vi "LVObject to JSON - Serializable Class - Returns JSON String.vi"() -> ()   [LabVIEW 2017, in "JSON Serializable Serializer Tests.lvlib"]
uses:
  JSON Serializable Serializer Tests.lvlib
  JSON Serializable Serializer/JSON Serializable Serializer.lvclass
  <vilib>/addons/_JKI Toolkits/Caraya/classes/Assert/Assert Equal Value_Variant.vi
  <vilib>/addons/_JKI Toolkits/Caraya/classes/Test/Test.lvclass
  <vilib>/addons/_JKI Toolkits/Caraya/classes/Assert/Assert.lvclass
  Mock JSON Serializable/Mock JSON Serializable.lvclass
panel:
  out "error out":errorcluster
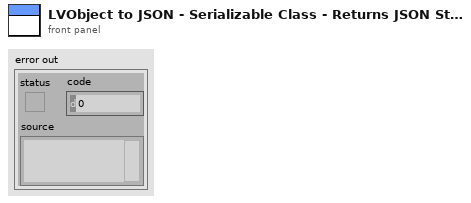
[diagram p1: front panel]
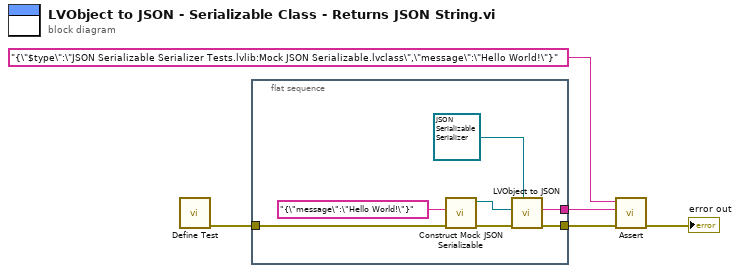
[diagram p0: block diagram]
diagram:
  n1 = call <vilib>:"Define Test.vi"() -> ("error out"=w3:errorcluster)  [unwired: 11 in]
  n2 = flat-sequence {
    tunnel: [w9] -> w5
    tunnel: [w10] -> w4
    tunnel: w3 -> [w11]
    frame #0 {
      n3 = call "Construct Mock JSON Serializable.vi"("error in (no error)"=w11, "To JSON <JSON> (\"{}\")"="{\"message\":\"Hello World!\"}" ("<JSON> (\"{}\")")) -> ("error out"=w8:errorcluster, "Mock JSON Serializable"=w7:refnum<class "Mock JSON Serializable.lvclass">)  [unwired: 8 in]
      n4 = call-dynamic "LVObject to JSON.vi"("JSON Serializable Serializer in"=refnum<class "JSON Serializable Serializer.lvclass"> refnum ("JSON Serializer.lvclass"), "error in (no error)"=w8, "Object"=w7) -> ("error out"=w10:errorcluster, "<JSON>Object"=w9:string)  [unwired: 7 in]
    }
  }
  n5 = call-poly <vilib>:"Assert.vi"("error in (no error)"=w4, "Y"=w5, "X"="{\"$type\":\"JSON Serializable Serializer Tests.lvlib:Mock JSON Serializable.lvclass\",\"message\":\"Hello World!\"}") -> ("error out"=→"error out":errorcluster)  [unwired: 8 in]
